vi "ap get protocol subversion.vi"(10 "dest_protocol_subversion":cluster{}, 11 "ap_handle":u32) -> (1 "function return":i32, 2 "dest_protocol_subversion out":cluster{}, 3 "ap_handle out":u32)   [LabVIEW 2019, in "apdm.lvlib"]
doc: "APDM_EXPORT int apdm_ap_get_protocol_subversion(apdm_ap_handle_t ap_handle, int64_t *dest_protocol_subversion);"
uses:
  apdm.lvlib
  Lee Lab/CP FES Walking 2018/Code/Working/LabVIEW/apdm.dll
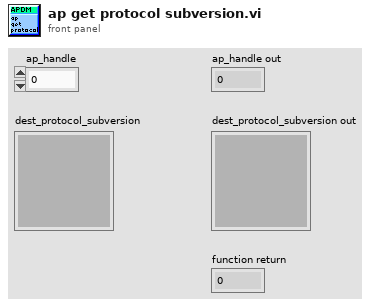
[diagram p1: front panel]
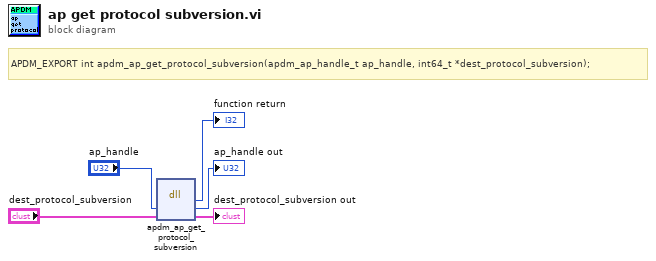
[diagram p0: block diagram]
diagram:
  # "APDM_EXPORT int apdm_ap_get_protocol_subversion(apdm_ap_handle_t ap_handle, int64_t *dest_protocol_subversion);"
  n1 = dll-call lib="C:/Users/jfalesi/Dropbox/Lee Lab/CP FES Walking 2018/Code/Working/LabVIEW/apdm.*" fn="apdm_ap_get_protocol_subversion"("ap_handle"="ap_handle", "dest_protocol_subversion"="dest_protocol_subversion") -> (→"function return":i32, "ap_handle"=→"ap_handle out":u32, "dest_protocol_subversion"=→"dest_protocol_subversion out":cluster{})  [unwired: 3 in, 2 out]
